vi "test_libssh2_channel_read.vi"() -> ()   [LabVIEW 2013, in "libssh2_integration_tests.lvlib"]
uses:
  libssh2_integration_tests.lvlib
  <vilib>/addons/_JKI Toolkits/Caraya/classes/Test/Test.lvclass
  libssh2/libssh2.lvlib
  <vilib>/addons/_JKI Toolkits/Caraya/classes/Assert/Assert.lvclass
panel:
  out "error out":errorcluster
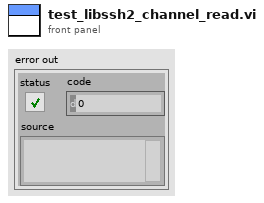
[diagram p1: front panel]
types:
  T1 = typedef "libssh2.lvlib/Session Refnum.ctl" = refnum<k1>
  T2 = typedef "libssh2.lvlib/Channel Refnum.ctl" = refnum<k1>
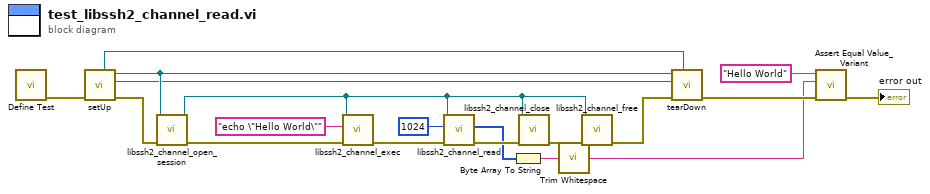
[diagram p0: block diagram]
diagram:
  n1 = call <vilib>:"Define Test.vi"() -> ("error out"=w18:errorcluster)  [unwired: 10 in, 1 out]
  n2 = call "setUp.vi"("error in (no error)"=w18) -> ("error out"=w13:errorcluster, "connection ID"=w14:refnum<k5>, "session"=w15:T1, "fixture"=w16:refnum<class "Server Fixture.lvclass">)  [unwired: 7 in]
  n3 = call "libssh2_channel_open_session.vi"("error in (no error)"=w13, "session"=w15) -> ("error out"=w10:errorcluster, "channel"=w7:T2)  [unwired: 8 in]
  n4 = call "libssh2_channel_exec.vi"("error in (no error)"=w10, "command"="echo \"Hello World\"", "channel"=w7) -> ("error out"=w9:errorcluster)  [unwired: 8 in]
  n5 = call "libssh2_channel_read.vi"("error in (no error)"=w9, "buffer length"=1024, "channel"=w7) -> ("error out"=w8:errorcluster, "buffer"=w4:u8[])  [unwired: 7 in]
  n6 = Byte Array To String(unsigned byte array=w4) -> (string=w3:string)
  n7 = call "libssh2_channel_close.vi"("error in (no error)"=w8, "channel"=w7) -> ("error out"=w5:errorcluster)  [unwired: 9 in]
  n8 = call <vilib>:"Trim Whitespace.vi"("string"=w3) -> ("trimmed string"=w2:string)  [unwired: 1 in]
  n9 = call "libssh2_channel_free.vi"("error in (no error)"=w5, "channel"=w7) -> ("error out"=w12:errorcluster)  [unwired: 9 in]
  n10 = call "tearDown.vi"("fixture"=w16, "error in (no error)"=w12, "connection ID"=w14, "session"=w15) -> ("error out"=w17:errorcluster)  [unwired: 7 in]
  n11 = call <vilib>:"Assert Equal Value_Variant.vi"("error in (no error)"=w17, "Y"=w2, "X"="Hello World") -> ("error out"=→"error out":errorcluster)  [unwired: 7 in, 1 out]
